vi "Merge Headers.vi"(6 "CloseAfterAdding [T]":bool=TRUE, 8 "error in (no error)":errorcluster, 10 "HTTPHeaders_NET to add":refnum<class "HttpHeaders_NET.lvclass">, 11 "HTTPHeaders_NET in":refnum<class "HttpHeaders_NET.lvclass">) -> (0 "error out":errorcluster, 3 "HTTPHeaders_NET out":refnum<class "HttpHeaders_NET.lvclass">)   [LabVIEW 2018, in "LabVIEWHTTPClient_NET.lvlib" / "HttpHeaders_NET.lvclass"]
uses:
  HttpHeaders_NET.lvclass
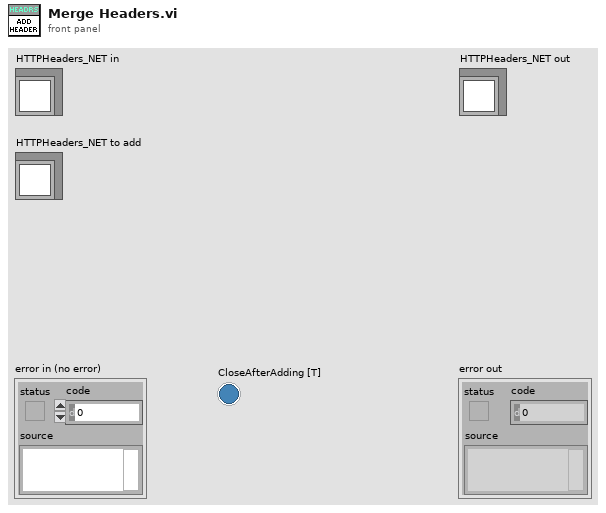
[diagram p1: front panel]
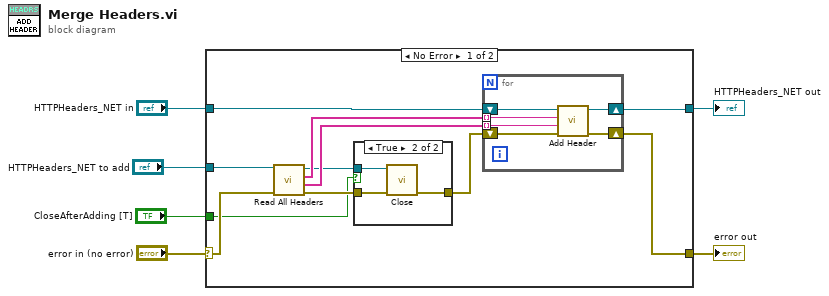
[diagram p0: block diagram]
diagram:
  n1 = case shown="No Error" "error in (no error)" {
    selector: "error in (no error)" -> [w11 w29]
    tunnel: [w8 w29] -> w5
    tunnel: [w15 w28] -> w3
    tunnel: "HTTPHeaders_NET in" -> [w16 w28]
    tunnel: "HTTPHeaders_NET to add" -> [w17 _]
    tunnel: "CloseAfterAdding [T]" -> [w7 _]
    frame No Error {
      n2 = call-dynamic "Read All Headers.vi"("error in (no error)"=w11, "HTTPHeaders_NET in"=w17) -> ("error out"=w10:errorcluster, "Header Values"=w13:string[], "Header Names"=w14:string[], "HTTPHeaders_NET out"=w12:refnum<class "HttpHeaders_NET.lvclass">)  [unwired: 6 in]
      n3 = case shown="True" w7 {
        tunnel: w12 -> [_ w27]
        tunnel: w10 -> [w24 w26]
        tunnel: [w24 w25] -> w9
        frame False {
        }
        frame True {
          n4 = call "Close.vi"("error in (no error)"=w26, "HTTPHeaders_NET in"=w27) -> ("error out"=w25:errorcluster)  [unwired: 9 in]
        }
      }
      n5 = for {
        tunnel: w14 -> [w18] mode=indexing
        tunnel: w13 -> [w21] mode=indexing
        shift-right: [w22] -> w15
        shift-left: w16 -> [w23]
        shift-right: [w19] -> w8
        shift-left: w9 -> [w20]
        n6 = call-dynamic "Add Header.vi"("error in (no error)"=w20, "Value"=w21, "Name"=w18, "HTTPHeaders_NET in"=w23) -> ("error out"=w19:errorcluster, "HTTPHeaders_NET out"=w22:refnum<class "HttpHeaders_NET.lvclass">)  [unwired: 6 in]
      }
    }
    frame Error {
    }
  }
  "error out" <- w5
  "HTTPHeaders_NET out" <- w3
